vi "Newport ITX-D3N ITHX Data.vi"(7 "Disable Filter?":bool=TRUE, 8 "error in (no error)":errorcluster, 11 "TCP Network Connection in":refnum<k5>) -> (0 "error out":errorcluster, 2 "ITHX Data":T1, 3 "TCP Network Connection out":refnum<k5>)   [LabVIEW 2023]
uses:
  Type Definitions/iBTHX Data Values.ctl
  Type Definitions/iTHX.ctl
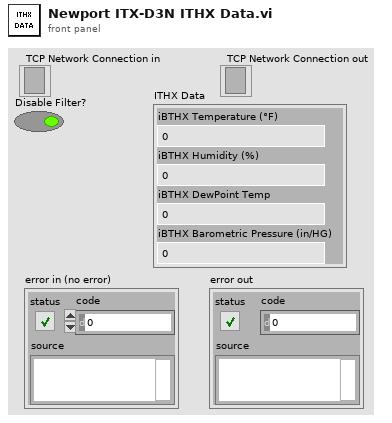
[diagram p1: front panel]
types:
  T1 = typedef "iBTHX Data Values.ctl" = cluster{"iBTHX Barometric Pressure (in/HG)":dbl, "iBTHX Humidity (%)":dbl, "iBTHX Temperature (°F)":dbl, "iBTHX DewPoint Temp":dbl}
  T2 = typedef "iTHX.ctl" = string
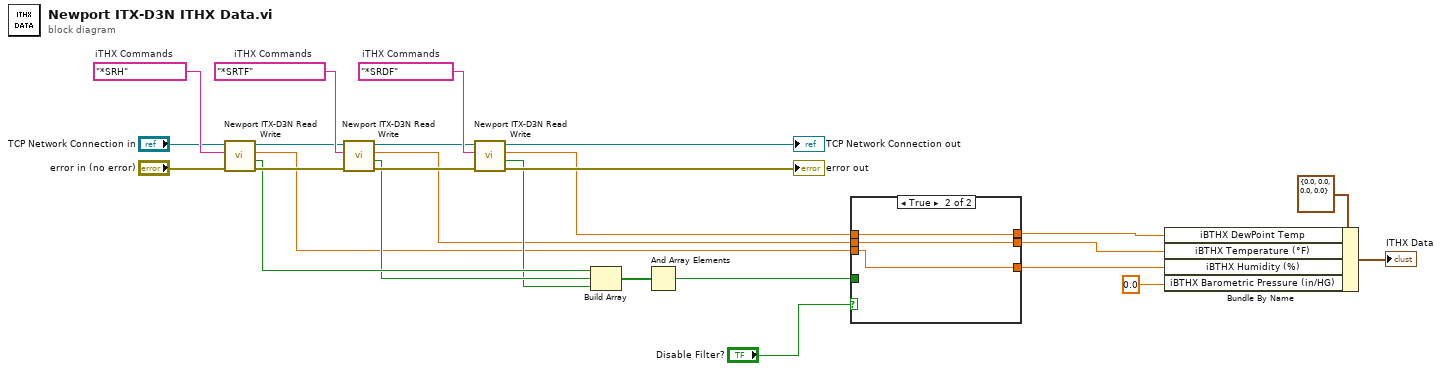
[diagram p0: block diagram]
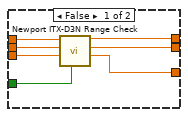
[diagram p2: hidden frame]
diagram:
  w26 = T2 "*SRDF"  # iTHX Commands
  w23 = T2 "*SRTF"  # iTHX Commands
  w20 = T2 "*SRH"  # iTHX Commands
  n1 = call "Newport ITX-D3N Read Write.vi"("error in (no error)"="error in (no error)", "iTHX Commands"=w20, "TCP Network Connection in"="TCP Network Connection in") -> ("error out"=w21:errorcluster, "In Range?"=w12:bool, "Output Data"=w5:dbl, "TCP Network Connection out"=w22:refnum<k5>)  [unwired: 5 in]
  n2 = call "Newport ITX-D3N Read Write.vi"("error in (no error)"=w21, "iTHX Commands"=w23, "TCP Network Connection in"=w22) -> ("error out"=w24:errorcluster, "In Range?"=w11:bool, "Output Data"=w7:dbl, "TCP Network Connection out"=w25:refnum<k5>)  [unwired: 5 in]
  n3 = call "Newport ITX-D3N Read Write.vi"("error in (no error)"=w24, "iTHX Commands"=w26, "TCP Network Connection in"=w25) -> ("error out"=→"error out":errorcluster, "In Range?"=w10:bool, "Output Data"=w8:dbl, "TCP Network Connection out"=→"TCP Network Connection out":refnum<k5>)  [unwired: 5 in]
  n4 = Build Array(w12, w11, w10) -> (w9:bool[])
  n5 = And Array Elements(Boolean array=w9) -> (logical AND=w6:bool)
  n6 = case shown="True" "Disable Filter?" {
    tunnel: w8 -> [w33 w36]
    tunnel: w7 -> [w32 w35]
    tunnel: w6 -> [w31 _]
    tunnel: w5 -> [w30 w34]
    tunnel: [w29 w36] -> w4
    tunnel: [w28 w35] -> w3
    tunnel: [w27 w34] -> w2
    frame False {
      n7 = call "Newport ITX-D3N Range Check.vi"("In Range?"=w31, "Humidity"=w30, "Temperature"=w32, "Dewpoint"=w33) -> ("Humidity Out"=w27:dbl, "Temperature Out"=w28:dbl, "Dewpoint Out"=w29:dbl)  [unwired: 3 in, 2 out]
    }
    frame True {
    }
  }
  n8 = Bundle By Name(cluster=T1 {"iBTHX Barometric Pressure (in/HG)"=0.0, "iBTHX Humidity (%)"=0.0, "iBTHX Temperature (°F)"=0.0, "iBTHX DewPoint Temp"=0.0} ("iBTHX"), "iBTHX DewPoint Temp"=w4, "iBTHX Temperature (°F)"=w3, "iBTHX Humidity (%)"=w2, "iBTHX Barometric Pressure (in/HG)"=0.0 ("iBTHX Barometric Pressure (mbar/hPa)")) -> (→"ITHX Data":T1)
